vi "clear chain.vi"(8 "error in (no error)":errorcluster, 11 "identifier":string) -> (0 "error out":errorcluster, 3 "function return":bool)   [LabVIEW 2015, in "XGL_DPP.lvlib"]
doc: "EXTERN DECLSPEC bool CALL_CONV clear_chain(const char* identifier);"
uses:
  XGL_DPP.lvlib
  XGL_DPP.dll
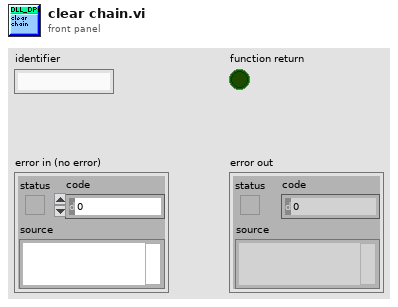
[diagram p1: front panel]
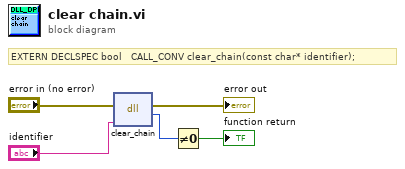
[diagram p0: block diagram]
diagram:
  # "EXTERN DECLSPEC bool   CALL_CONV clear_chain(const char* identifier);"
  n1 = dll-call lib="D:/Users/XRF/Desktop/Dante_acquire4/libs/Dante/XGL_DPP.*" fn="clear_chain"(error in="error in (no error)", "identifier"="identifier") -> (error out=→"error out":errorcluster, "return type"=w4:u8)  [unwired: 3 in, 1 out]
  n2 = Not Equal To 0?(x=w4) -> (x != 0?=→"function return":bool)
